vi "Create Enum Type Specialization.vi"(7 "error in (no error)":errorcluster, 9 "Parameter Name":string, 10 "Enum reference in":refnum<vi>) -> (0 "error out":errorcluster, 2 "Parameter Type Specialization Output":T1, 3 "Control reference out":refnum<vi>)   [LabVIEW 2020, in "MeasurementLink Measurement Server.lvlib"]
uses:
  MeasurementLink Measurement Server.lvlib
  TypeDefs/Parameter Type Specialization.ctl
  TypeDefs/Type Specialization.ctl
  TypeDefs/Type Specialization Key.ctl
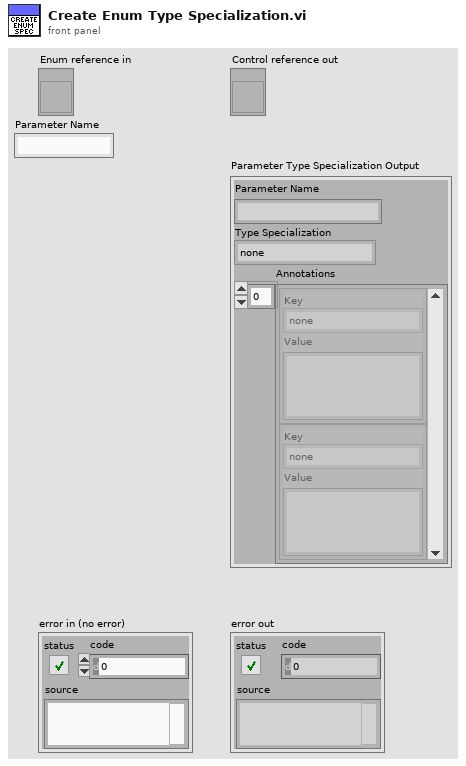
[diagram p1: front panel]
types:
  T1 = typedef "MeasurementLink Measurement Server.lvlib/Parameter Type Specialization.ctl" = cluster{"Parameter Name":string, "Type Specialization":T2, "Annotations":cluster{"Key":T3, "Value":string}[]}
  T2 = typedef "MeasurementLink Measurement Server.lvlib/Type Specialization.ctl" = enum16{"none", "pin", "path", "enum"}
  T3 = typedef "MeasurementLink Measurement Server.lvlib/Type Specialization Key.ctl" = enum16{"none", "pin.instrument_type", "enum.values"}
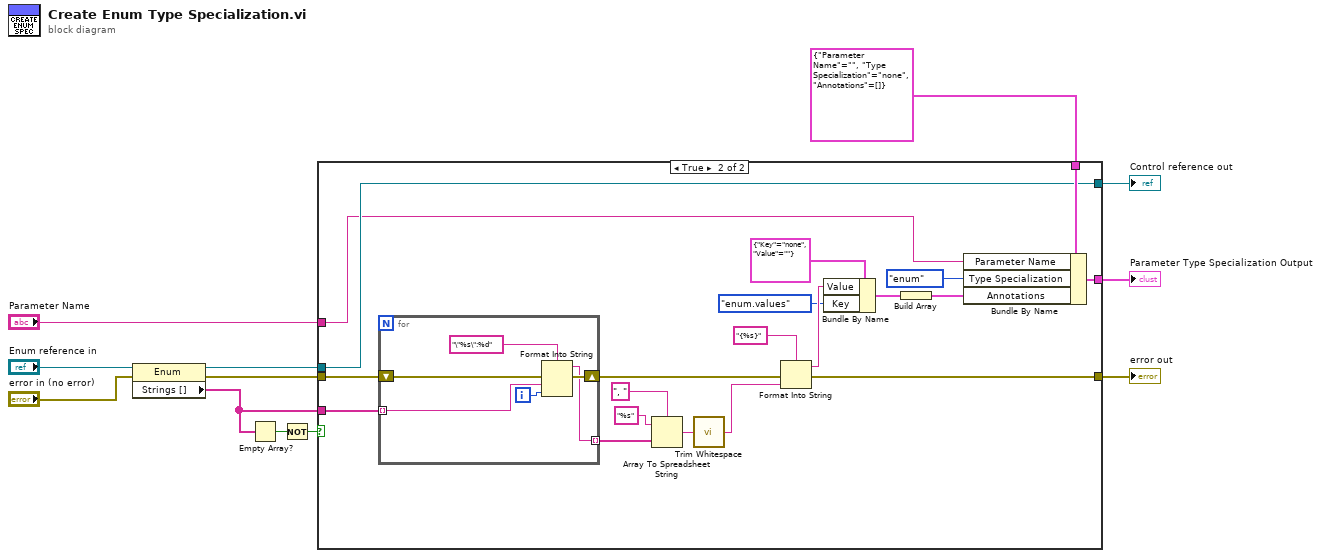
[diagram p0: block diagram]
diagram:
  n1 = property class="Enum"(reference="Enum reference in", error in="error in (no error)") -> (reference out=w4:refnum<vi>, error out=w3:errorcluster, "Strings []"=w2:string[])
  n2 = Empty Array?(array=w2) -> (empty?=w8:bool)
  n3 = Not(x=w8) -> (.not. x?=w7:bool)
  n4 = case shown="True" w7 {
    tunnel: [w15 w34] -> w12
    tunnel: T1 {"Parameter Name"="", "Type Specialization"=enum."none", "Annotations"=[]} ("Parameter Type Specialization Input") -> [w15 w32]
    tunnel: [w14 w27] -> w10
    tunnel: w2 -> [_ w19]
    tunnel: w4 -> [w13 w18]
    tunnel: [w13 w18] -> w9
    tunnel: w3 -> [w14 w17]
    tunnel: "Parameter Name" -> [_ w16]
    frame False {
    }
    frame True {
      n5 = for {
        tunnel: w19 -> [w40] mode=indexing
        shift-right: [w38] -> w28
        shift-left: w17 -> [w37]
        tunnel: [w36] -> w22 mode=indexing
        i -> [w39]
        n6 = Format Into String(format string="\"%s\":%d", error in=w37, w40, w39) -> (resulting string=w36:string, error out=w38:errorcluster)  [unwired: 1 in]
      }
      n7 = Array To Spreadsheet String(delimiter (Tab)=", ", array=w22, 3:"%s" ("format string")) -> (spreadsheet string=w21:string)
      n8 = call <vilib>:"Trim Whitespace.vi"("string"=w21) -> ("trimmed string"=w20:string)  [unwired: 1 in]
      n9 = Format Into String(format string="{%s}", error in=w28, w20) -> (resulting string=w30:string, error out=w27:errorcluster)  [unwired: 1 in]
      n10 = Bundle By Name(cluster=cluster{"Key":T3, "Value":string} {"Key"=enum."none", "Value"=""} ("input cluster"), "Value"=w30, "Key"=Type_Specialization_Key."enum.values") -> (w25:cluster{"Key":T3, "Value":string})
      n11 = Build Array(w25) -> (w26:cluster{"Key":T3, "Value":string}[])
      n12 = Bundle By Name(cluster=w32, "Parameter Name"=w16, "Type Specialization"=Type_Specialization."enum", "Annotations"=w26) -> (w34:T1)
    }
  }
  "error out" <- w10
  "Parameter Type Specialization Output" <- w12
  "Control reference out" <- w9
